vi "ConfigCore.vi"(8 "Error In":errorcluster, 10 "ConfigAIn":refnum<class "ConfigA.lvclass">, 11 "RefIn":refnum<class "IReference.lvclass">) -> (0 "Error Out":errorcluster, 2 "ConfigAOut":refnum<class "ConfigA.lvclass">, 3 "RefOut":refnum<class "IReference.lvclass">)   [LabVIEW 2019, in "ConfigA.lvclass"]
uses:
  ConfigA.lvclass
  IReference/IReference.lvclass
  DMM/DMM.lvclass
  C:/Repo/LabVIEW-SOLID-Examples/Architecture/IReference/IReference.lvclass
  ConfigA.lvclass/ConfigA.ctl
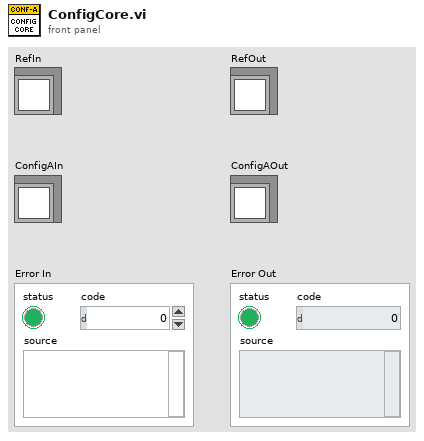
[diagram p1: front panel]
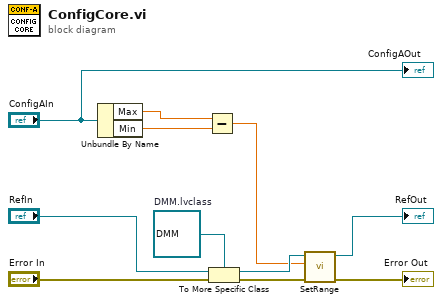
[diagram p0: block diagram]
diagram:
  w7 = refnum<class "DMM.lvclass"> refnum  # DMM.lvclass
  n1 = Unbundle By Name("ConfigAIn") -> ("Max"=w11:dbl, "Min"=w10:dbl)
  n2 = Subtract(x=w11, y=w10) -> (x-y=w3:dbl)
  n3 = To More Specific Class(target class=w7, reference="RefIn", error in="Error In") -> (specific class reference=w5:refnum<class "DMM.lvclass">, error out=w6:errorcluster)
  n4 = call "SetRange.vi"("Error In"=w6, "Range"=w3, "DMMIn"=w5) -> ("Error Out"=→"Error Out":errorcluster, "DMMOut"=→"RefOut":refnum<class "DMM.lvclass">)  [unwired: 7 in]
  "ConfigAOut" <- "ConfigAIn"
